vi "nonlinear magnet location fit.vi"(7 "board inverted?":bool, 8 "fixed parameters":T1={"x magnet"=nan, "y magnet"=nan, "z magnet"=nan, "Br*V (T*mm^3)"=nan, "theta - moment angle to z-axis"=nan, "phi - moment angle to x-axis"=nan}, 10 "Magnetometer reading set":T2, 11 "initial parameters":T1) -> (0 "residue":dbl, 2 "fit OK":bool, 3 "fit parameters":T1)   [LabVIEW 2017]
uses:
  typedefs/magnet location fit result.ctl
  typedefs/magnetomter reading set.ctl
  <vilib>/gmath/NumericalOptimization/Nonlinear Curve Fit LM bound.vi
  <vilib>/gmath/NI_Gmath.lvlib
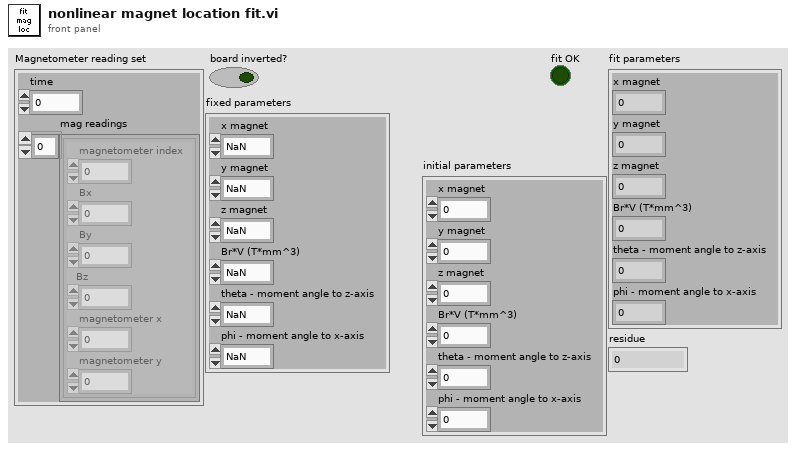
[diagram p1: front panel]
types:
  T1 = typedef "magnet location fit result.ctl" = cluster{"x magnet":dbl, "y magnet":dbl, "z magnet":dbl, "Br*V (T*mm^3)":dbl, "theta - moment angle to z-axis":dbl, "phi - moment angle to x-axis":dbl}
  T2 = typedef "magnetomter reading set.ctl" = cluster{"time":fxp<+,48,48>, "mag readings":cluster{"magnetometer index":dbl, "Bx":dbl, "By":dbl, "Bz":dbl, "magnetometer x":dbl, "magnetometer y":dbl}[]}
  T3 = cluster{"parameter minimum":dbl[], "parameter maximum":dbl[]}
  T4 = cluster{"best fit parameters[0]":dbl, "best fit parameters[1]":dbl, "best fit parameters[2]":dbl, "best fit parameters[3]":dbl, "best fit parameters[4]":dbl, "best fit parameters[5]":dbl}
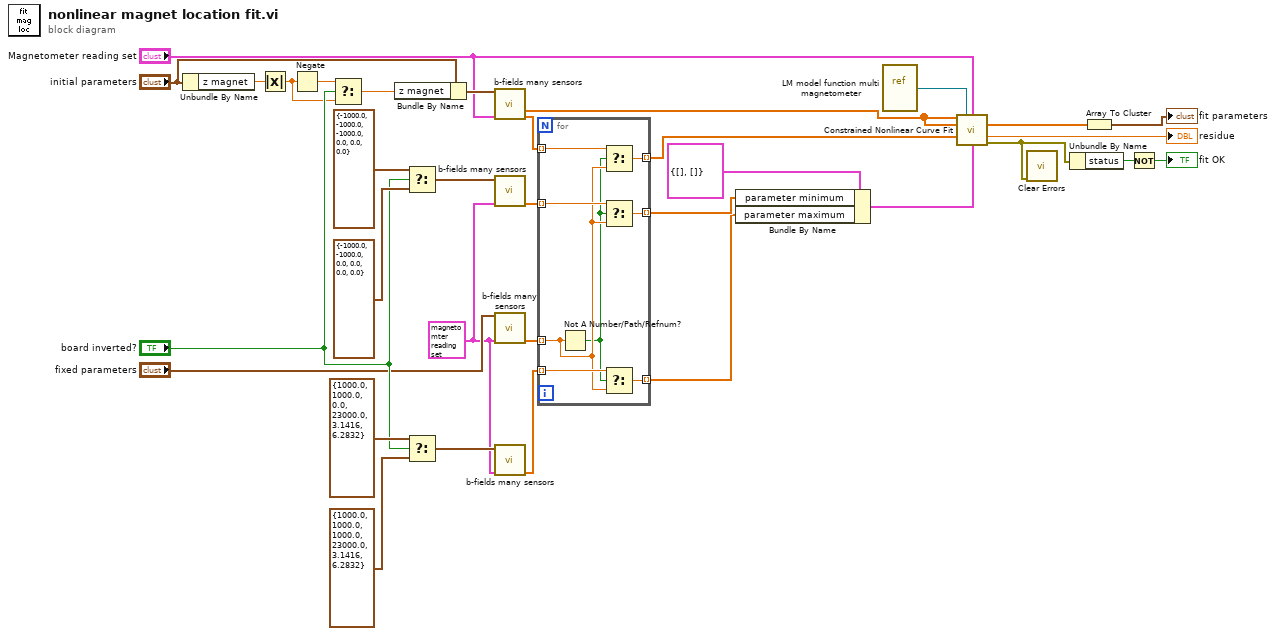
[diagram p0: block diagram]
diagram:
  w8 = T2 {"time"=0.0, "mag readings"=[]} ("Magnetometer reading set")
  n1 = Unbundle By Name("initial parameters") -> ("z magnet"=w21:dbl)
  n2 = Absolute Value(x=w21) -> (abs(x)=w19:dbl)
  n3 = Negate(x=w19) -> (-x=w18:dbl)
  n4 = Select(t=w18, s="board inverted?", f=w19) -> (s? t:f=w16:dbl)
  n5 = Bundle By Name(cluster="initial parameters", "z magnet"=w16) -> (w17:T1)
  n6 = Select(t=T1 {"x magnet"=-1000.0, "y magnet"=-1000.0, "z magnet"=-1000.0, "Br*V (T*mm^3)"=0.0, "theta - moment angle to z-axis"=0.0, "phi - moment angle to x-axis"=0.0} ("initial parameters 2"), s="board inverted?", f=T1 {"x magnet"=-1000.0, "y magnet"=-1000.0, "z magnet"=0.0, "Br*V (T*mm^3)"=0.0, "theta - moment angle to z-axis"=0.0, "phi - moment angle to x-axis"=0.0} ("initial parameters 2")) -> (s? t:f=w27:T1)
  n7 = Select(t=T1 {"x magnet"=1000.0, "y magnet"=1000.0, "z magnet"=0.0, "Br*V (T*mm^3)"=23000.0, "theta - moment angle to z-axis"=3.1416, "phi - moment angle to x-axis"=6.2832} ("initial parameters 2"), s="board inverted?", f=T1 {"x magnet"=1000.0, "y magnet"=1000.0, "z magnet"=1000.0, "Br*V (T*mm^3)"=23000.0, "theta - moment angle to z-axis"=3.1416, "phi - moment angle to x-axis"=6.2832} ("initial parameters 2")) -> (s? t:f=w24:T1)
  n8 = call "b-fields many sensors.vi"("magnet location params"=w17, "Magnetometer reading set"="Magnetometer reading set") -> ("mf - flat"=w31:dbl[], "param vector out"=w2:dbl[])  [unwired: 7 in, 5 out]
  n9 = call "b-fields many sensors.vi"("magnet location params"=w27, "Magnetometer reading set"=w8) -> ("param vector out"=w7:dbl[])  [unwired: 7 in, 6 out]
  n10 = call "b-fields many sensors.vi"("magnet location params"="fixed parameters", "Magnetometer reading set"=w8) -> ("param vector out"=w5:dbl[])  [unwired: 7 in, 6 out]
  n11 = call "b-fields many sensors.vi"("magnet location params"=w24, "Magnetometer reading set"=w8) -> ("param vector out"=w6:dbl[])  [unwired: 7 in, 6 out]
  n12 = for {
    tunnel: w7 -> [w39] mode=indexing
    tunnel: w6 -> [w41] mode=indexing
    tunnel: w5 -> [w36] mode=indexing
    tunnel: [w40] -> w3 mode=indexing
    tunnel: [w38] -> w4 mode=indexing
    tunnel: w2 -> [w37] mode=indexing
    tunnel: [w34] -> w1 mode=indexing
    n13 = Not A Number/Path/Refnum?(number/path/refnum=w36) -> (NaN/Path/Refnum?=w35:bool)
    n14 = Select(t=w37, s=w35, f=w36) -> (s? t:f=w34:dbl)
    n15 = Select(t=w39, s=w35, f=w36) -> (s? t:f=w38:dbl)
    n16 = Select(t=w41, s=w35, f=w36) -> (s? t:f=w40:dbl)
  }
  n17 = Bundle By Name(cluster=T3 {"parameter minimum"=[], "parameter maximum"=[]} ("parameter bounds"), "parameter minimum"=w4, "parameter maximum"=w3) -> (w23:T3)
  n18 = vi-ref "LM model function multi magnetometer.vi"() -> (w32:refnum<vi>)
  n19 = call-poly <vilib>:"Constrained Nonlinear Curve Fit.vi"("Y"=w31, "f(x,a)"=w32, "data"="Magnetometer reading set", "X"=w31, "initial parameters"=w1, "parameter bounds"=w23) -> ("best fit parameters"=w15:dbl[], "residue"=→"residue":dbl, "error out"=w13:errorcluster)  [unwired: 4 in, 3 out]
  n20 = call <vilib>:"Clear Errors.vi"("error in (no error)"=w13) -> ()  [unwired: 5 in, 2 out]
  n21 = Unbundle By Name(w13) -> ("status"=w14:bool)
  n22 = Array To Cluster(array=w15) -> (cluster=→"fit parameters":T4)
  n23 = Not(x=w14) -> (.not. x?=→"fit OK":bool)
